vi "Write Axis Map.vi"(8 "error in (no error)":errorcluster, 10 "Axis Map":map{string, T1}(c390), 11 "Motion Controller in":refnum<class "Motion Controller.lvclass">) -> (0 "error out":errorcluster, 3 "Motion Controller out":refnum<class "Motion Controller.lvclass">)   [LabVIEW 2022 SP3, in "Motion Controller.lvclass"]
uses:
  Motion Controller.lvclass
  Motion Controller.lvclass/Motion Controller.ctl
  Axis Parameters.ctl
  Axis Settings.ctl
  Axis Data.ctl
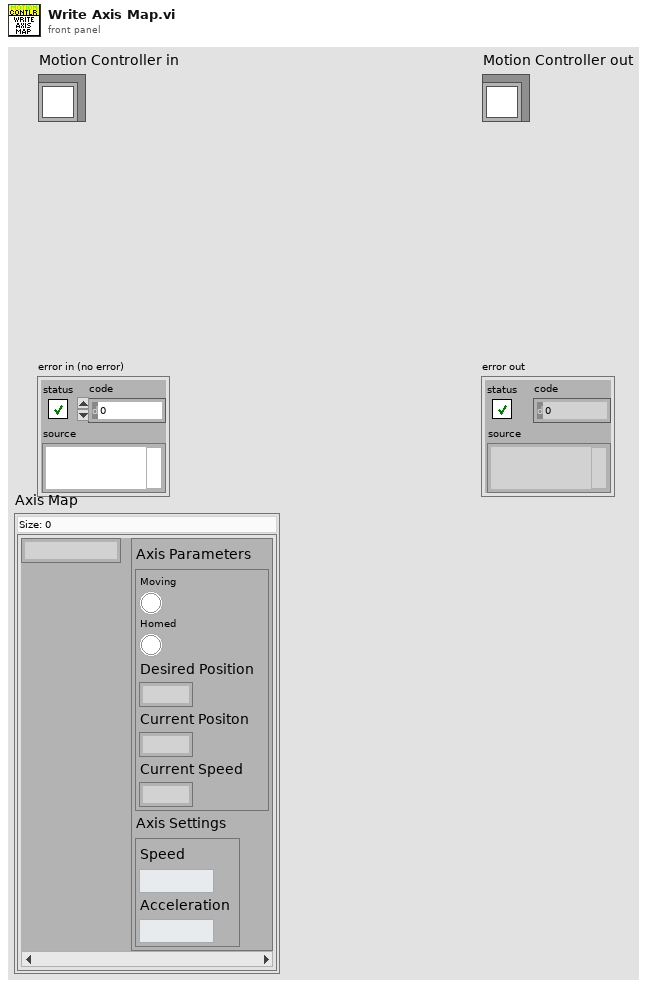
[diagram p1: front panel]
types:
  T1 = typedef "Motion Controller.lvclass/Axis Data.ctl" = cluster{"Axis Parameters":T2, "Axis Settings":T3}
  T2 = typedef "Motion Controller.lvclass/Axis Parameters.ctl" = cluster{"Moving":bool, "Homed":bool, "Desired Position":dbl, "Current Positon":dbl, "Current Speed":dbl}
  T3 = typedef "Motion Controller.lvclass/Axis Settings.ctl" = cluster{"Speed":dbl, "Acceleration":dbl}
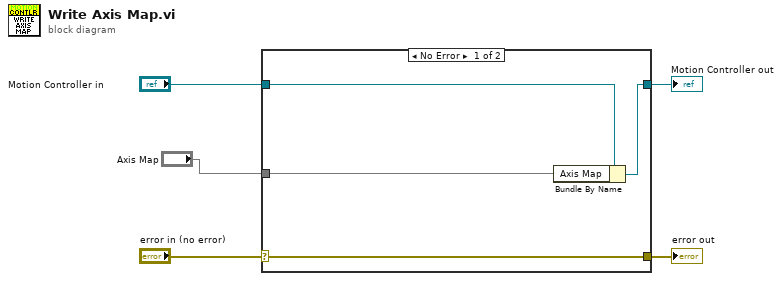
[diagram p0: block diagram]
diagram:
  n1 = case shown="No Error" "error in (no error)" {
    selector: "error in (no error)" -> [w9 w10]
    tunnel: [w9 w10] -> w4
    tunnel: [w7 w11] -> w2
    tunnel: "Motion Controller in" -> [w8 w11]
    tunnel: "Axis Map" -> [w6 _]
    frame No Error {
      n2 = Bundle By Name(cluster=w8, "Axis Map"=w6) -> (w7:refnum<class "Motion Controller.lvclass">)
    }
    frame Error {
    }
  }
  "error out" <- w4
  "Motion Controller out" <- w2
